vi "Evaluate.vi"(7 "Variables":refnum<class "Variables.lvclass">, 8 "error in (no error)":errorcluster, 9 "Sequence Time":T1, 11 "Condition in":refnum<class "Condition.lvclass">) -> (0 "error out":errorcluster, 2 "Result":bool, 3 "Condition out":refnum<class "Condition.lvclass">)   [LabVIEW 2020, in "VolatusSeq.lvlib" / "Condition.lvclass"]
uses:
  Condition.lvclass
  Sequence Time.ctl
  Variables/Variables.lvclass
  Condition.lvclass/Condition.ctl
  VolatusSeq.lvlib
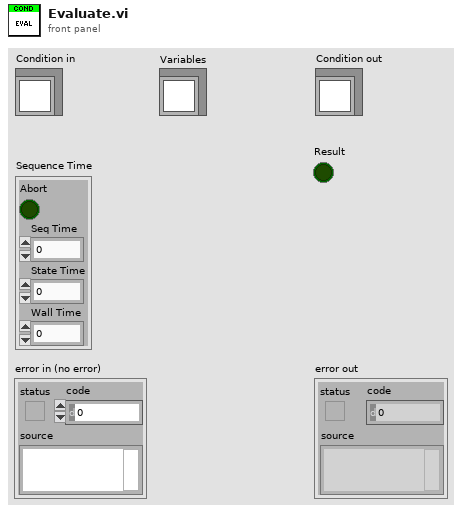
[diagram p1: front panel]
types:
  T1 = typedef "VolatusSeq.lvlib/Sequence Time.ctl" = cluster{"Abort":bool, "Seq Time":dbl, "State Time":dbl, "Wall Time":dbl}
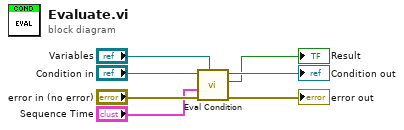
[diagram p0: block diagram]
diagram:
  n1 = call-dynamic "Eval Condition.vi"("Variables"="Variables", "error in (no error)"="error in (no error)", "Sequence Time"="Sequence Time", "Condition in"="Condition in") -> ("error out"=→"error out":errorcluster, "Result"=→"Result":bool, "Condition out"=→"Condition out":refnum<class "Condition.lvclass">)  [unwired: 5 in]
